vi "Refill.vi"(0 "object in":refnum<class "CetoniPump.lvclass">, 1 "refill rate":dbl, 2 "index":i32, 5 "error in (no error)":errorcluster) -> (14 "object out":refnum<class "CetoniPump.lvclass">, 19 "error out":errorcluster)   [LabVIEW 2023, in "CetoniPump.lvclass"]
uses:
  CetoniPump.lvclass
  CetoniPump.lvclass/CetoniPump.ctl
  CETONI_SDK/lib/labview/labbCAN_Pump_API/labbCAN_Pump_API.lvlib
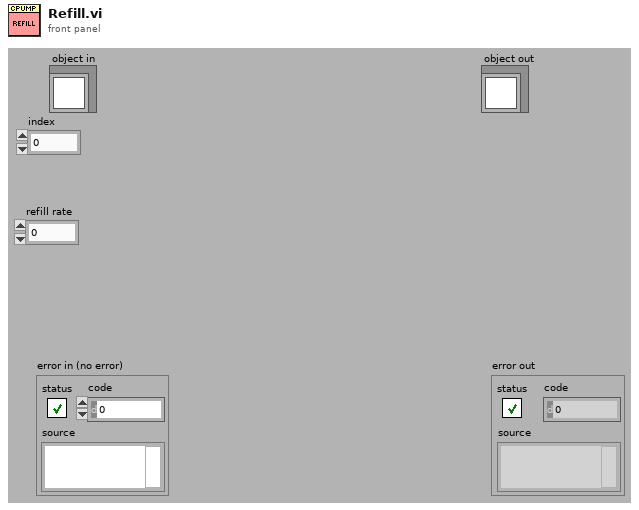
[diagram p1: front panel]
types:
  T1 = cluster{"Pump Handle":i64, "Pump Name":string, "Maximum Volume":dbl, "Maximum Flow Rate":dbl, "Flow Rate":dbl, "Target Level":dbl, "Valve Handle":i64, "Has Valve?":bool, "Actual valve position":i32}[]
  T2 = cluster{"Pump Handle":i64, "Pump Name":string, "Maximum Volume":dbl, "Maximum Flow Rate":dbl, "Flow Rate":dbl, "Target Level":dbl, "Valve Handle":i64, "Has Valve?":bool, "Actual valve position":i32}
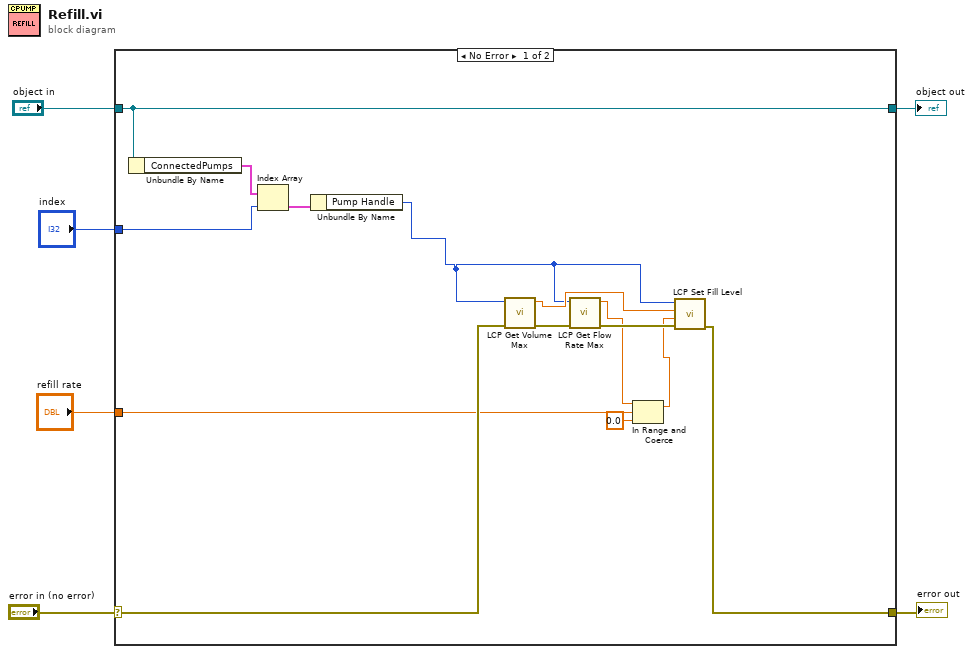
[diagram p0: block diagram]
diagram:
  n1 = case shown="No Error" "error in (no error)" {
    selector: "error in (no error)" -> [w16 w22]
    tunnel: [w15 w22] -> w5
    tunnel: [w20 w21] -> w3
    tunnel: "object in" -> [w20 w21]
    tunnel: "index" -> [w11 _]
    tunnel: "refill rate" -> [w8 _]
    frame No Error {
      n2 = Unbundle By Name(w20) -> ("ConnectedPumps"=w14:T1)
      n3 = Index Array(array=w14, index=w11) -> (element=w13:T2)
      n4 = Unbundle By Name(w13) -> ("Pump Handle"=w12:i64)
      n5 = call "LCP Get Volume Max.vi"("error in (no error)"=w16, "Pump Handle"=w12) -> ("error out"=w19:errorcluster, "Maximum Volume"=w17:dbl)  [unwired: 8 in]
      n6 = call "LCP Get Flow Rate Max.vi"("error in (no error)"=w19, "Pump Handle"=w12) -> ("error out"=w18:errorcluster, "Maximum Flow Rate"=w10:dbl)  [unwired: 8 in]
      n7 = In Range and Coerce(upper limit=w10, x=w8, lower limit=0.0) -> (coerced(x)=w9:dbl)  [unwired: 1 out]
      n8 = call "LCP Set Fill Level.vi"("error in (no error)"=w18, "Flow"=w9, "Level"=w17, "Pump Handle"=w12) -> ("error out"=w15:errorcluster)  [unwired: 7 in]
    }
    frame Error {
    }
  }
  "error out" <- w5
  "object out" <- w3
